vi "excelcolumnconcat.vi"() -> ()   [LabVIEW 2020]
uses:
  <vilib>/addons/_office/excel.llb/Excel Get Data ([dbl]).vi
  <vilib>/Utility/file.llb/Write To Spreadsheet File (DBL).vi
  <vilib>/Utility/NIReport.llb/NI_report.lvclass
  <vilib>/Utility/NIReport.llb/Excel/NI_Excel.lvclass
  <vilib>/addons/_office/NI_ReportGenerationToolkit.lvlib
panel:
  in  "error in (no error)":errorcluster caption="entrée d'erreur (pas d'erreur)"
  in  "precission":string="6"
  out "Numer of sheet":i32=120
  in  "end (66, 3)":cluster{"row":i32, "column":i32}={"row"=66, "column"=3}
  in  "start (2,0)":cluster{"row":i32, "column":i32}={"row"=2, "column"=0}
  in  "Destination path":path=path "C:/Users/lab user/Desktop/cm"
  in  "output file name":string="aaa.xls"
  in  "Select Column No.(-1)":i32=3
  out "Selected Column":ext[](array[numeric])=[3.90764143958222e-05, 7.61822884669527e-05, 0.000114766080514528, 0.000154096182086505, 0.000194036736502312, 0.000211308521102183, 0.000244270893745124, 0.000280356936855242, 0.000316674588248134, 0.000346021261066198, 0.000431595311965793, 0.000475546228699386, 0.00051031302427873, 0.000549825024791062, 0.000611612165812403, 0.000633780786301941, 0.000619862112216651, 0.000508421915583313, 0.000282114429865032, 0.000305013061733916, 0.000323792832205072, 0.000337357050739229, 0.000354817893821746, 0.00036767779965885, 0.0004547196731437, 0.000476125016575679, 0.000460526207461953, 0.000503468560054898, 0.000534854829311371, 0.000561434135306627, 0.000575784360989928, 0.000602852320298553, 0.00058649032143876, 0.000528524222318083, 0.00047412229469046, 0.000426320446422324, 0.000394057540688664, 0.00035078008659184, 0.000306837755488232, 0.00027094132383354, 0.000238187931245193, 0.000209086530958302, 0.000183560623554513, 0.000159952367539518, 0.000138665272970684, 0.000119993324915413, 0.000103645805211272, 8.89317743713036e-05, 7.6019176049158e-05, 6.45195468678139e-05, 5.44001304660924e-05, 4.54942346550524e-05, 3.67294742318336e-05, 3.00935225823196e-05, 2.41571360675152e-05, 1.92496518138796e-05, 1.50192872752086e-05, 1.14403846964706e-05, 8.30091448733583e-06, 5.93545382798766e-06, 4.11274368161685e-06, 2.75384900305653e-06, 1.63597394475801e-06, 7.48674267470051e-07, 1.28115464903544e-08] format="%#_6e"
  in  "Select Excel file":path=path "C:/Users/lab user/Desktop/cm/D8-RESET-4.xls"
  out "Output Added Columns":ext[][](array[numeric]) format="%#_6e"
  out "Sheet Values":ext[][](array[numeric]) format="%_6e"
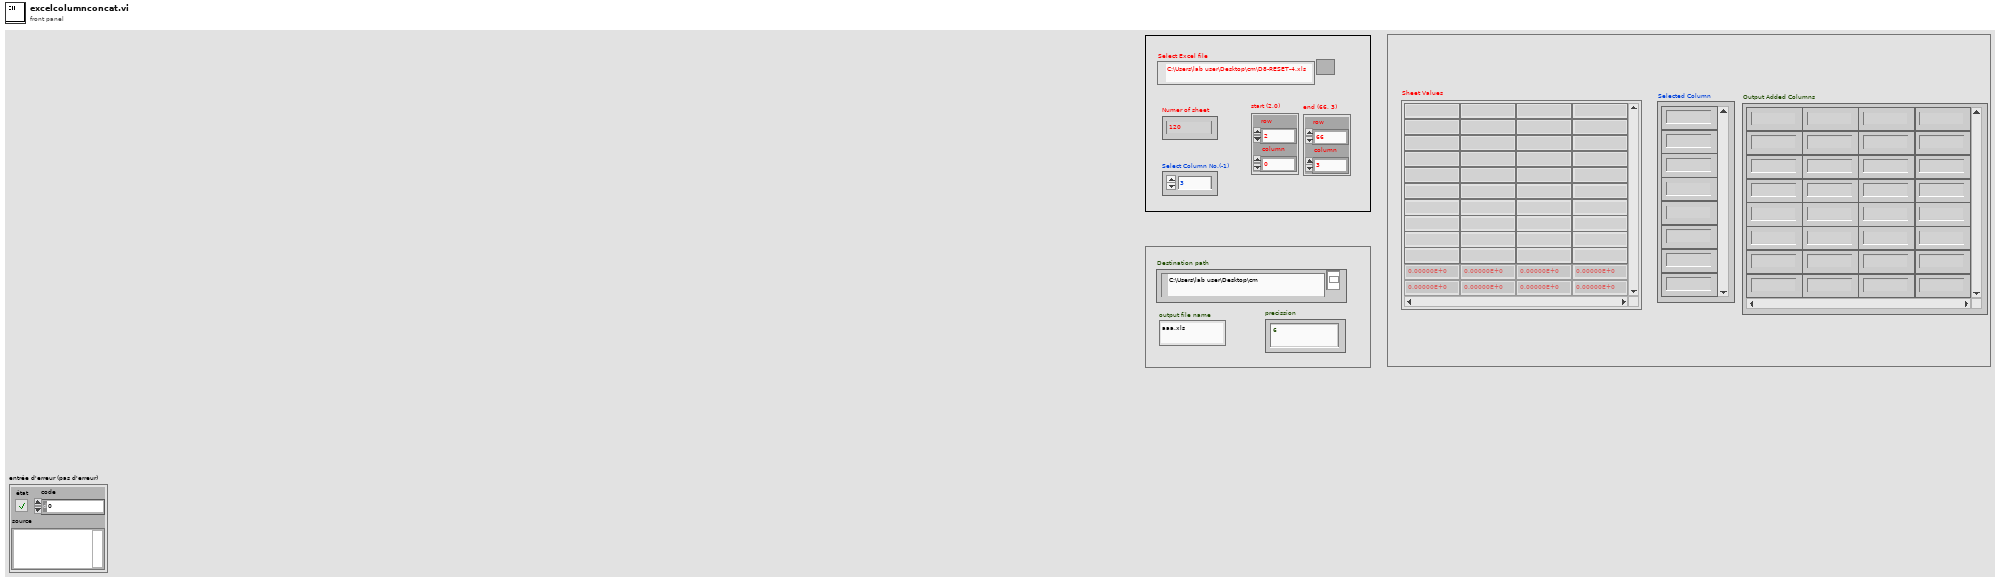
[diagram p1: front panel]
types:
  T1 = enum16{"Standard Report", "HTML", "Word", "Excel"}
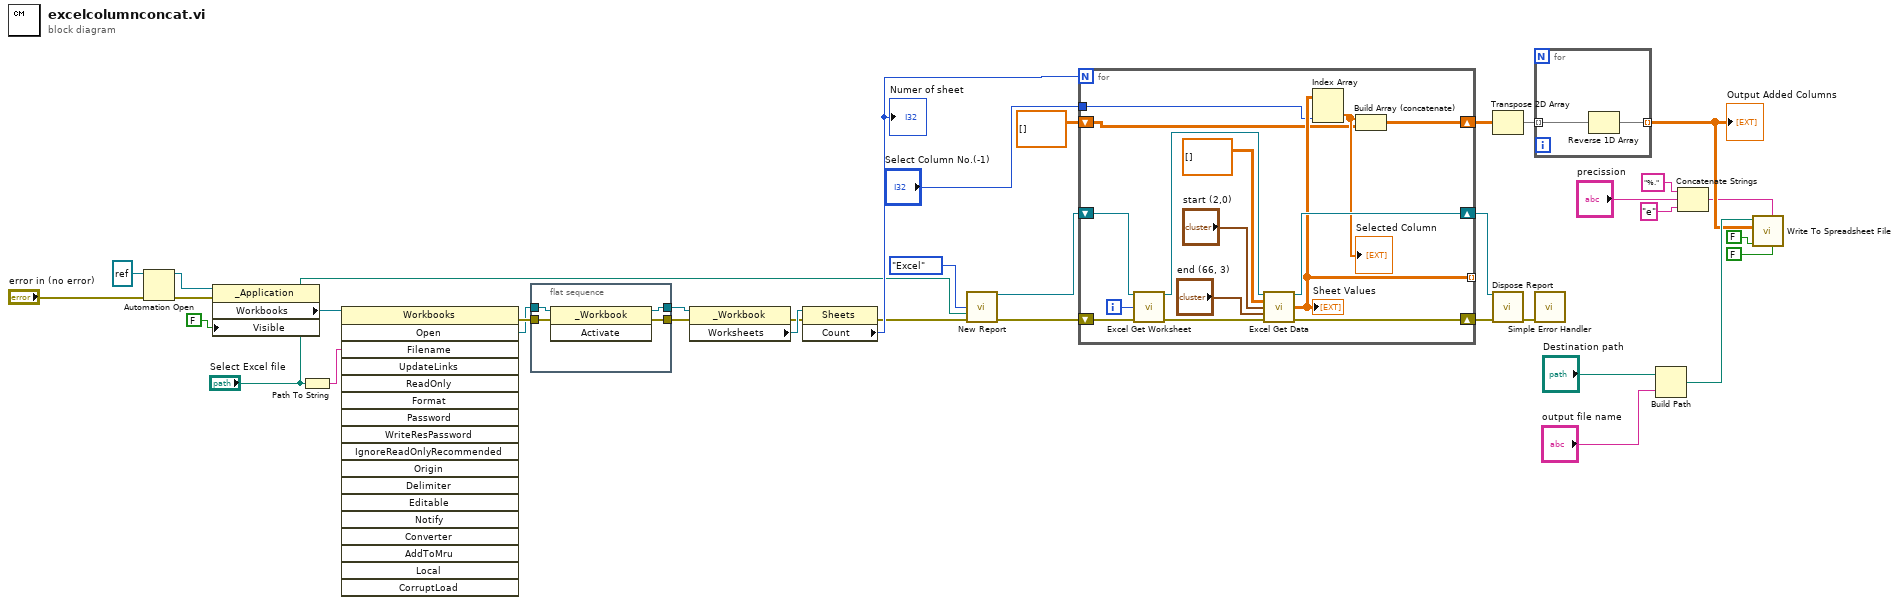
[diagram p0: block diagram]
diagram:
  n1 = Automation Open(error in (no error)="error in (no error)", Automation Refnum=refnum<k7> refnum ("Excel._Application")) -> (Automation Refnum=w15:refnum<k7>, error out=w14:errorcluster)  [unwired: 2 in]
  n2 = property on="Nœud de propriété" class="_Application"(reference=w15, error in=w14, "Visible"=FALSE) -> ("Workbooks"=w10:refnum<k7>)  [unwired: 2 out]
  n3 = Path To String(path="Select Excel file") -> (string=w12:string)
  n4 = invoke class="Workbooks" method="Open"(reference=w10, "Filename"=w12) -> (error out=w11:errorcluster, "Open"=w9:refnum<k7>)  [unwired: 16 in, 16 out]
  n5 = flat-sequence {
    tunnel: w11 -> [w40]
    tunnel: w9 -> [w39]
    tunnel: [w38] -> w8
    tunnel: [w37] -> w7
    frame #0 {
      n6 = invoke class="_Workbook" method="Activate"(reference=w39, error in=w40) -> (reference out=w38:refnum<k7>, error out=w37:errorcluster)  [unwired: 1 in, 1 out]
    }
  }
  n7 = property class="_Workbook"(reference=w8, error in=w7) -> (error out=w3:errorcluster, "Worksheets"=w4:refnum<k7>)  [unwired: 1 out]
  n8 = property class="Sheets"(reference=w4, error in=w3) -> (error out=w2:errorcluster, "Count"=w6:i32)  [unwired: 1 out]
  "Numer of sheet" <- w6
  n9 = call <vilib>:"New Report.vi"("report type"=T1."Excel", "template (empty)"="Select Excel file", "error in (no error)"=w2) -> ("report out"=w36:refnum<class "NI_report.lvclass">, "error out"=w35:errorcluster)  [unwired: 11 in]
  n10 = for {
    N: w6 -> [_]
    shift-right: [w50] -> w34
    shift-left: w36 -> [w55]
    shift-right: [w49] -> w33
    shift-left: w35 -> [w54]
    tunnel: [w47] -> _ mode=indexing
    shift-right: [w44] -> w32
    shift-left: ext[][] [] -> [w45]
    tunnel: "Select Column No.(-1)" -> [w43]
    i -> [w48]
    n11 = call <vilib>:"Excel Get Worksheet.vi"("report in"=w55, "worksheet index (0)"=w48, "error in (no error)"=w54) -> ("report out"=w52:refnum<class "NI_report.lvclass">, "error out"=w53:errorcluster)  [unwired: 11 in]
    n12 = call-poly <vilib>:"Excel Get Data.vi"("report in"=w52, "data type"=ext[][] [], "start (-1, -1)"="start (2,0)", "end (-1, -1)"="end (66, 3)", "error in (no error)"=w53) -> ("report out"=w50:refnum<class "NI_report.lvclass">, "data"=w47:ext[][], "error out"=w49:errorcluster)  [unwired: 8 in]
    "Sheet Values" <- w47
    n13 = Index Array(array=w47, index (col)=w43) -> (element=w46:ext[])  [unwired: 1 in]
    "Selected Column" <- w46
    n14 = Build Array (concatenate)(w46, w45) -> (w44:ext[][])
  }
  n15 = Transpose 2D Array(2D array=w32) -> (transposed array=w30:ext[][])
  n16 = call-dynamic "Dispose Report.vi"("report in"=w34, "error in (no error)"=w33) -> ("error out"=w1:errorcluster)  [unwired: 13 in]
  n17 = for {
    tunnel: w30 -> [w57] mode=indexing
    tunnel: [w56] -> w23 mode=indexing
    n18 = Reverse 1D Array(array=w57) -> (reversed array=w56:ext[])
  }
  "Output Added Columns" <- w23
  n19 = call <vilib>:"Simple Error Handler.vi"("error in (no error)"=w1) -> ()  [unwired: 4 in, 5 out]
  n20 = Build Path(base path="Destination path", name or relative path="output file name") -> (appended path=w24:path)
  n21 = Concatenate Strings("%.", "precission", "e") -> (w18:string)
  n22 = call-poly <vilib>:"Write To Spreadsheet File.vi"("transpose? (no:F)"=FALSE, "format (%.3f)"=w18, "append to file? (new file:F)"=FALSE, "2D data"=w23, "file path (dialog if empty)"=w24) -> ()  [unwired: 3 in, 1 out]
